vi "ArduinoEdgesense.vi"(4 "Error In":errorcluster, 6 "Temperature Progression IN":T1, 7 "Ref. No.":u32) -> (0 "Error Out":errorcluster, 1 "Z [µm]":i32, 2 "Temperature Progression OUT":T1, 3 "Temperature [°C]":dbl)   [LabVIEW 2013]
uses:
  global/ProbeStation.vi
  InstrControl/ArduinoControl/ArduinoControl.lvclass
  InstrControl/InstrumentSetup.vi
  InstrControl/InstrControl.lvclass
  <vilib>/ErrorRing/Error Ring.xnode
  <vilib>/Utility/error.llb/Error Cluster From Error Code.vi
  InstrControl/ProbeStationControl/ProbeStationControl.lvclass
panel:
  out "dZ [µm]":i32
  out "previous Z [µm]":i32
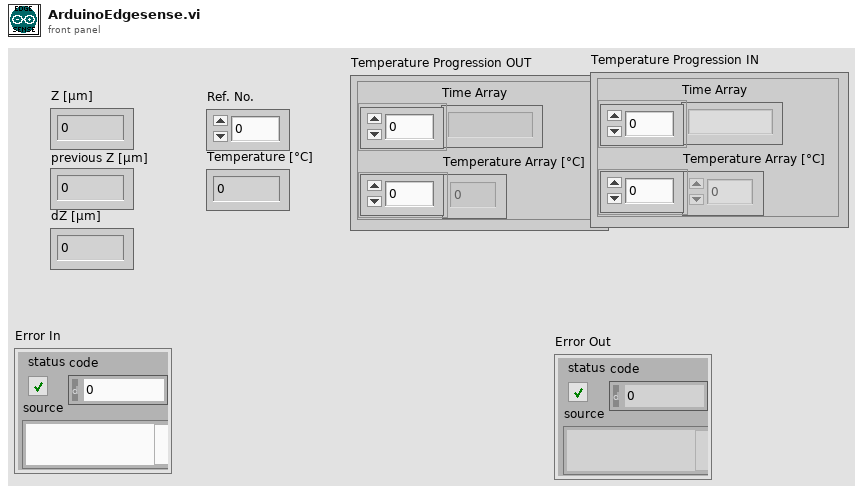
[diagram p1: front panel]
types:
  T1 = cluster{"Time Array":string[], "Temperature Array [°C]":dbl[]}
  T2 = cluster{"initial Z [µm]":i32, "search band [µm]":i32, "speed [µm/step]":i32, "overdrive [µm]":i32}
  T3 = cluster{"VISA address":refnum<visa-resource-name>, "T sensor":enum16{"SHT", "DS"}, "Arduino":refnum<class "ArduinoControl.lvclass">}
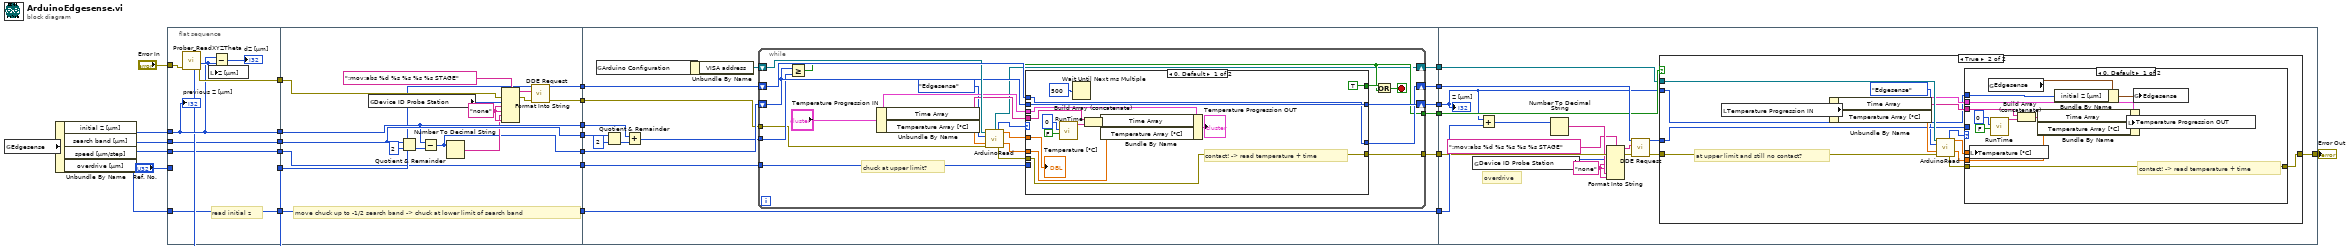
[diagram p0: block diagram]
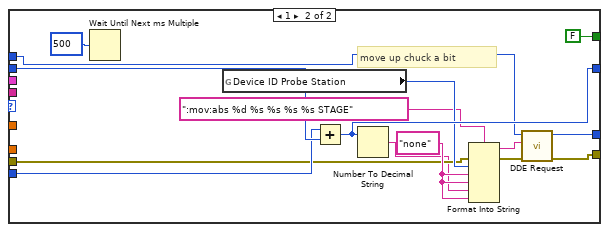
[diagram p2: hidden frame]
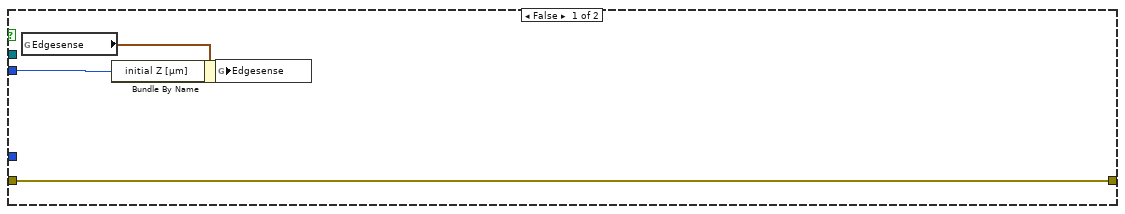
[diagram p3: hidden frame]
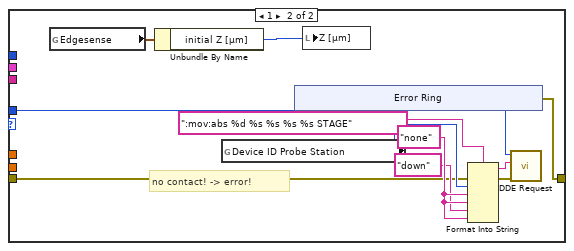
[diagram p4: hidden frame]
diagram:
  n1 = global read "ProbeStation.vi" "Edgesense"() -> (w27:T2)
  n2 = Unbundle By Name(w27) -> ("initial Z [µm]"=w26:i32, "search band [µm]"=w25:i32, "speed [µm/step]"=w24:i32, "overdrive [µm]"=w23:i32)
  n3 = flat-sequence {
    tunnel: w26 -> [w32]
    tunnel: w25 -> [w30]
    tunnel: w24 -> [w29]
    tunnel: w23 -> [w28]
    tunnel: "Ref. No." -> [w31]
    tunnel: "Error In" -> [w36]
    tunnel: [w32] -> w19
    tunnel: [w30] -> w18
    tunnel: [w29] -> w17
    tunnel: [w28] -> w16
    tunnel: [w35] -> w15
    tunnel: [w31] -> w14
    tunnel: w19 -> [w50]
    tunnel: w18 -> [w53]
    tunnel: w17 -> [w39]
    tunnel: w16 -> [w38]
    tunnel: w15 -> [w47]
    tunnel: w14 -> [w40]
    tunnel: [w50] -> w13
    tunnel: [w53] -> w12
    tunnel: [w39] -> w11
    tunnel: [w38] -> w10
    tunnel: [w37] -> w9
    tunnel: [w41] -> w8
    tunnel: [w42] -> w7
    tunnel: w13 -> [w61]
    tunnel: w12 -> [w62]
    tunnel: w11 -> [w69]
    tunnel: w10 -> [w55]
    tunnel: w9 -> [w70]
    tunnel: w8 -> [w68]
    tunnel: w7 -> [w54]
    tunnel: [w55] -> w6
    tunnel: [w67] -> w5
    tunnel: [w59] -> w4
    tunnel: [w58] -> w3
    tunnel: [w57] -> w2
    tunnel: [w56] -> w1
    tunnel: [w124] -> w20
    tunnel: w6 -> [w136]
    tunnel: w5 -> [w134]
    tunnel: w4 -> [w125]
    tunnel: w3 -> [w135]
    tunnel: w2 -> [w121]
    tunnel: w1 -> [w123]
    frame #0 {
      # "read initial z"
      n4 = call-dynamic "Prober_ReadXYZTheta.vi"("Theta location [mdeg]"=w31, "error in (no error)"=w36) -> ("error out"=w35:errorcluster, "Z location [µm]"=w33:i32)  [unwired: 5 in, 3 out]
      n5 = local write "Z [µm]"(w33) -> ()
      n6 = Subtract(x=w32, y=w33) -> (x-y=→"dZ [µm]":i32)
      "previous Z [µm]" <- w32
    }
    frame #1 {
      w49 = "none"
      # "move chuck up to -1/2 search band -> chuck at lower limit of search band"
      n7 = global read "ProbeStation.vi" "Device ID Probe Station"() -> (w48:i32)
      n8 = Quotient & Remainder(x=w53, y=2) -> (floor(x/y)=w51:i32)  [unwired: 1 out]
      n9 = Subtract(x=w50, y=w51) -> (x-y=w37:i32)
      n10 = Number To Decimal String(number=w37) -> (decimal integer string=w45:string)  [unwired: 1 in]
      n11 = Format Into String(format string=":mov:abs %d %s %s %s %s STAGE", error in=w47, w48, w49, w49, w45, w49) -> (resulting string=w44:string, error out=w43:errorcluster)  [unwired: 1 in]
      n12 = call <vilib>:"DDE Request.vi"("error in (no error)"=w43, "item"=w44, "conversation refnum in"=w40) -> ("error out"=w42:errorcluster, "conversation refnum out"=w41:u32)  [unwired: 4 in, 1 out]
    }
    frame #2 {
      n13 = global read "InstrumentSetup.vi" "Arduino Configuration"() -> (w66:T3)
      n14 = Quotient & Remainder(x=w62, y=2) -> (floor(x/y)=w64:i32)  [unwired: 1 out]
      n15 = Add(x=w61, y=w64) -> (x+y=w60:i32)
      n16 = Unbundle By Name(w66) -> ("VISA address"=w65:refnum<visa-resource-name>)
      n17 = while {
        shift-right: [w90] -> w57
        shift-left: w70 -> [w84]
        tunnel: w69 -> [w91]
        tunnel: [w87] -> w67
        shift-right: [w71] -> w56
        shift-left: w65 -> [w86]
        tunnel: w60 -> [w83]
        shift-right: [w76] -> w58
        shift-left: w68 -> [w89]
        tunnel: [w75] -> w59
        tunnel: w54 -> [w73]
        stop <- w81 stop-if-true
        # "chuck at upper limit?"
        n18 = Greater Or Equal?(x=w84, y=w83) -> (x >= y?=w75:bool)
        n19 = Unbundle By Name("Temperature Progression IN") -> ("Time Array"=w79:string[], "Temperature Array [°C]"=w80:dbl[])
        n20 = call "ArduinoRead.vi"("VISA resource name"=w86, "interlock or edgesense"=enum16{"Interlock", "Edgesense", "Humidity"}."Edgesense", "Temperature IN"=w80, "error in (no error)"=w73) -> ("VISA resource name OUT"=w71:refnum<visa-resource-name>, "Edgesense Status"=w88:u16, "Temperature [°C]"=w77:dbl, "Temperature OUT"=w78:dbl[], "error out"=w85:errorcluster)  [unwired: 4 in, 3 out]
        n21 = case shown="0, Default" w88 {
          tunnel: w84 -> [w105 w119]
          tunnel: w91 -> [_ w118]
          tunnel: [w105 w117] -> w90
          tunnel: w89 -> [w95 w107]
          tunnel: [w98 w110] -> w87
          tunnel: [TRUE FALSE] -> w82
          tunnel: w85 -> [w98 w109]
          tunnel: "Temperature Progression IN" -> [w103 _]
          tunnel: w79 -> [w100 _]
          tunnel: w78 -> [w97 _]
          tunnel: w77 -> [w96 _]
          tunnel: [w95 w106] -> w76
          frame 0, Default {
            # "contact! -> read temperature + time"
            n22 = call "RunTime.vi"("Probing done - new estimation"=FALSE, "Flag"=0) -> ("Time so far"=w93:string)  [unwired: 2 in, 3 out]
            n23 = Wait Until Next ms Multiple(millisecond multiple=500) -> ()  [unwired: 1 out]
            n24 = Build Array (concatenate)(w100, w93) -> (w99:string[])
            n25 = Bundle By Name(cluster=w103, "Time Array"=w99, "Temperature Array [°C]"=w97) -> (→"Temperature Progression OUT":T1)
            "Temperature [°C]" <- w96
          }
          frame 1 {
            w115 = "none"
            # "move up chuck a bit"
            n26 = Wait Until Next ms Multiple(millisecond multiple=500) -> ()  [unwired: 1 out]
            n27 = global read "ProbeStation.vi" "Device ID Probe Station"() -> (w114:i32)
            n28 = Add(x=w118, y=w119) -> (x+y=w117:i32)
            n29 = Number To Decimal String(number=w117) -> (decimal integer string=w108:string)  [unwired: 1 in]
            n30 = Format Into String(format string=":mov:abs %d %s %s %s %s STAGE", error in=w109, w114, w115, w115, w108, w115) -> (resulting string=w112:string, error out=w111:errorcluster)  [unwired: 1 in]
            n31 = call <vilib>:"DDE Request.vi"("error in (no error)"=w111, "item"=w112, "conversation refnum in"=w107) -> ("error out"=w110:errorcluster, "conversation refnum out"=w106:u32)  [unwired: 4 in, 1 out]
          }
        }
        n32 = Or(x=w82, y=w75) -> (x .or. y?=w81:bool)
      }
    }
    frame #3 {
      w128 = "none"
      # "overdrive"
      n33 = global read "ProbeStation.vi" "Device ID Probe Station"() -> (w129:i32)
      n34 = Add(x=w121, y=w136) -> (x+y=w127:i32)
      n35 = Number To Decimal String(number=w127) -> (decimal integer string=w133:string)  [unwired: 1 in]
      n36 = Format Into String(format string=":mov:abs %d %s %s %s %s STAGE", error in=w134, w129, w128, w128, w133, w128) -> (resulting string=w131:string, error out=w132:errorcluster)  [unwired: 1 in]
      n37 = call <vilib>:"DDE Request.vi"("error in (no error)"=w132, "item"=w131, "conversation refnum in"=w135) -> ("error out"=w126:errorcluster, "conversation refnum out"=w122:u32)  [unwired: 4 in, 1 out]
      n38 = case shown="True" w125 {
        tunnel: w126 -> [w140 w153]
        tunnel: [w140 w146] -> w124
        tunnel: w123 -> [_ w151]
        tunnel: w122 -> [_ w144]
        tunnel: w121 -> [w137 w142]
        frame False {
          n39 = global read "ProbeStation.vi" "Edgesense"() -> (w139:T2)
          n40 = Bundle By Name(cluster=w139, "initial Z [µm]"=w137) -> (w138:T2)
          n41 = global write "ProbeStation.vi" "Edgesense"(w138) -> ()
        }
        frame True {
          # "at upper limit and still no contact?"
          n42 = local read "Temperature Progression IN"() -> (w149:T1)
          n43 = Unbundle By Name(w149) -> ("Time Array"=w143:string[], "Temperature Array [°C]"=w152:dbl[])
          n44 = call "ArduinoRead.vi"("VISA resource name"=w151, "interlock or edgesense"=enum16{"Interlock", "Edgesense", "Humidity"}."Edgesense", "Temperature IN"=w152, "error in (no error)"=w153) -> ("Edgesense Status"=w147:u16, "Temperature [°C]"=w148:dbl, "Temperature OUT"=w150:dbl[], "error out"=w145:errorcluster)  [unwired: 4 in, 4 out]
          n45 = case shown="0, Default" w147 {
            tunnel: w150 -> [w164 _]
            tunnel: w149 -> [w162 _]
            tunnel: w148 -> [w161 _]
            tunnel: [w160 w169] -> w146
            tunnel: w145 -> [w160 w170]
            tunnel: w144 -> [_ w172]
            tunnel: w143 -> [w159 _]
            tunnel: w142 -> [w154 _]
            frame 0, Default {
              # "contact! -> read temperature + time"
              n46 = local write "Temperature [°C]"(w161) -> ()
              n47 = global read "ProbeStation.vi" "Edgesense"() -> (w155:T2)
              n48 = call "RunTime.vi"("Probing done - new estimation"=FALSE, "Flag"=0) -> ("Time so far"=w158:string)  [unwired: 2 in, 3 out]
              n49 = Build Array (concatenate)(w159, w158) -> (w165:string[])
              n50 = Bundle By Name(cluster=w162, "Time Array"=w165, "Temperature Array [°C]"=w164) -> (w163:T1)
              n51 = Bundle By Name(cluster=w155, "initial Z [µm]"=w154) -> (w156:T2)
              n52 = local write "Temperature Progression OUT"(w163) -> ()
              n53 = global write "ProbeStation.vi" "Edgesense"(w156) -> ()
            }
            frame 1 {
              w174 = "none"
              # "no contact! -> error!"
              n54 = global read "ProbeStation.vi" "Edgesense"() -> (w168:T2)
              n55 = Unbundle By Name(w168) -> ("initial Z [µm]"=w167:i32)
              n56 = global read "ProbeStation.vi" "Device ID Probe Station"() -> (w175:i32)
              n57 = xnode "Error Ring"() -> ("error out"=w169:errorcluster)
              n58 = local write "Z [µm]"(w167) -> ()
              n59 = Format Into String(format string=":mov:abs %d %s %s %s %s STAGE", error in=w170, w175, w174, w174, "down", w174) -> (resulting string=w173:string, error out=w177:errorcluster)  [unwired: 1 in]
              n60 = call <vilib>:"DDE Request.vi"("error in (no error)"=w177, "item"=w173, "conversation refnum in"=w172) -> ()  [unwired: 4 in, 3 out]
            }
          }
        }
      }
      "Z [µm]" <- w121
    }
  }
  "Error Out" <- w20
